vi "Generate Reference Waveforms.vi"(6 "reset phase":bool, 8 "error in (no error)":errorcluster, 11 "Generator in":refnum<class "Generator.lvclass">) -> (0 "error out":errorcluster, 1 "REF_Y":waveform(dbl)[](array[waveform]), 2 "REF_X":waveform(dbl)[](array[waveform]), 3 "Generator out":refnum<class "Generator.lvclass">, 4 "phase reset":bool)   [LabVIEW 2019, in "Generator.lvclass"]
uses:
  Generator.lvclass
  typedefs/REF.Channel--Cluster.ctl
  Generator.lvclass/Generator.ctl
  <vilib>/measure/NI_MABase.lvlib
  Waveform.Attributes/Waveform.Attributes.lvlib
panel:
  in  "Tab Control":enum32{"Page 1", "Graph"}(tab)
  out "sampling info":cluster{"Fs":dbl, "#s":dbl}={"Fs"=1000.0, "#s"=1000.0} {"Fs" format="%.2p"}
  out "REF Channels":T1[](array[typedef]) {"TC" min=1.0; "Phase" min=0.0001 format="%#_3p"; "Frequency" format="%.3g"; "Channel" min=1 max=10000 format="%.3g"}
  out "Waveform Graph":waveform(dbl)[](graph)
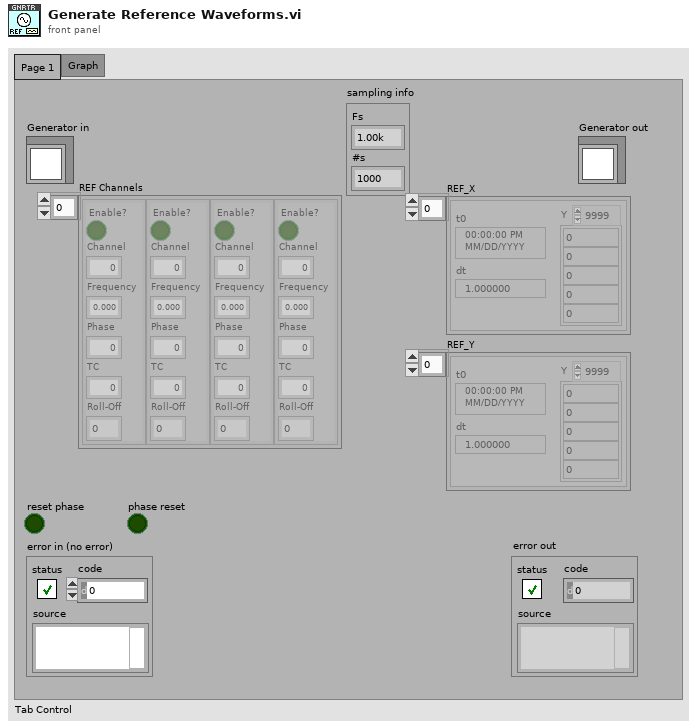
[diagram p1: front panel]
types:
  T1 = typedef "Generator.lvclass/REF.Channel--Cluster.ctl" = cluster{"Enable?":bool, "Channel":i32, "Frequency":dbl, "Phase":dbl, "TC":dbl, "Roll-Off":i32}
  T2 = typedef "Generator.lvclass/REF.Channel--Cluster--Array.ctl" = T1[]
  T3 = typedef "Generator.lvclass/Sampling--Cluster.ctl" = cluster{"Fs":dbl, "#s":dbl}
  T4 = enum16{"Sine Wave", "Triangle Wave", "Square Wave", "Sawtooth Wave"}
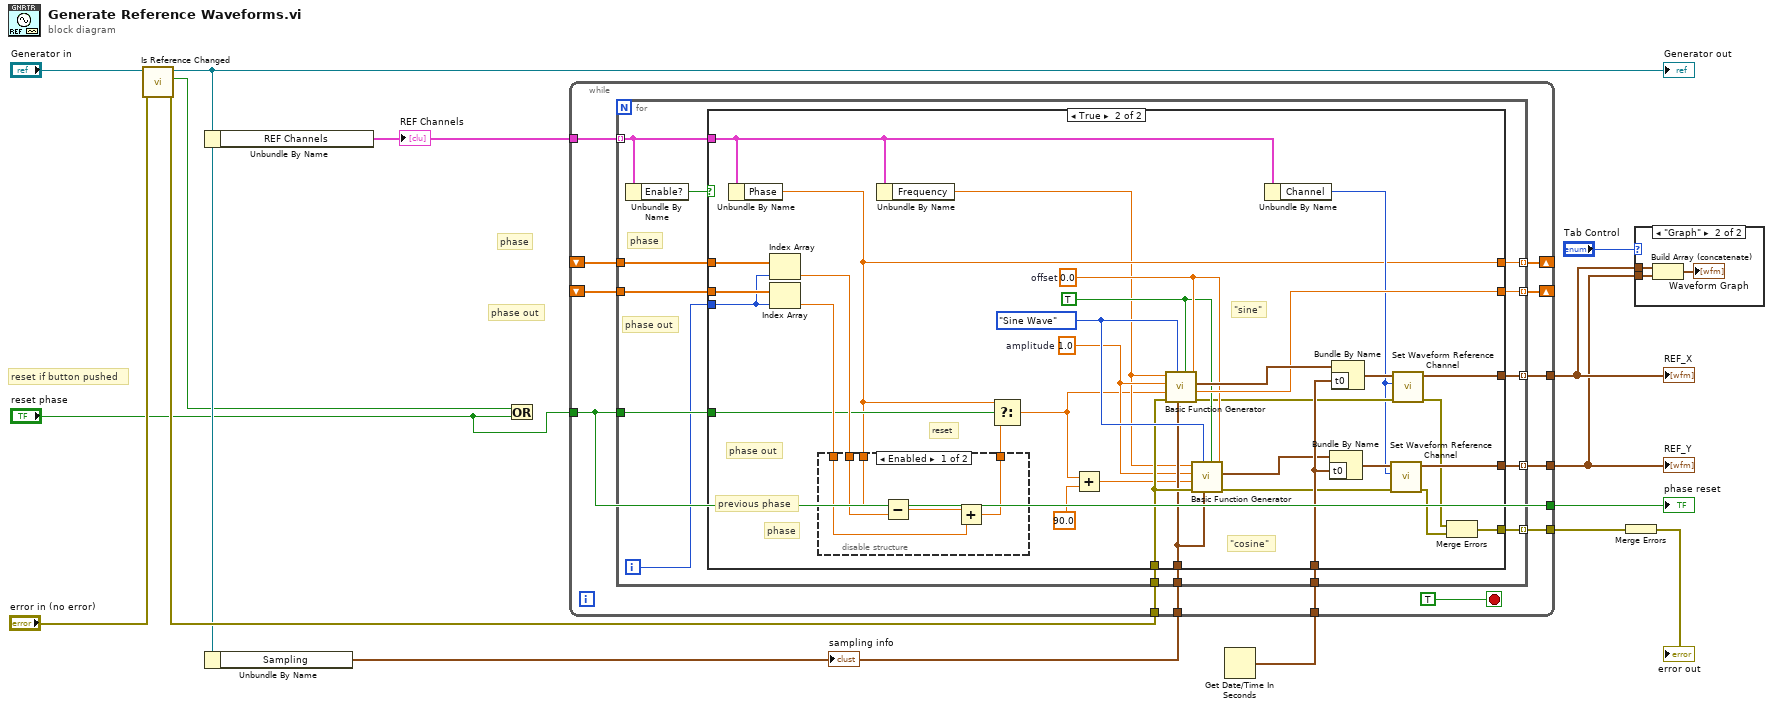
[diagram p0: block diagram]
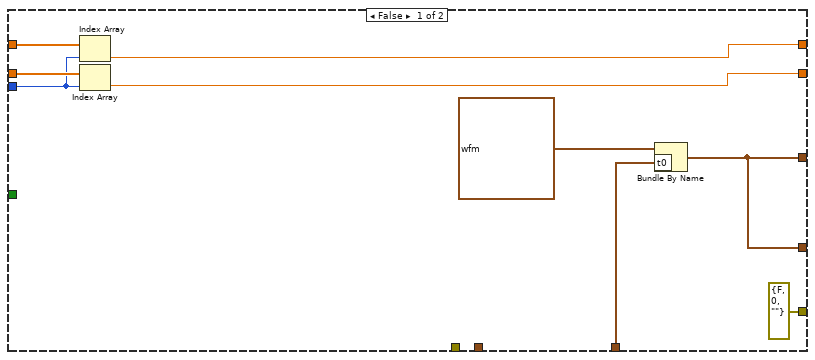
[diagram p2: hidden frame]
diagram:
  # "reset if button pushed"
  # "phase out"
  # "phase"
  n1 = call "Is Reference Changed.vi"("error in (no error)"="error in (no error)", "Generator in"="Generator in") -> ("error out"=w12:errorcluster, "REF frequency or phase changed?"=w3:bool, "Generator out"=w4:refnum<class "Generator.lvclass">)  [unwired: 7 in]
  "Generator out" <- w4
  n2 = Unbundle By Name(w4) -> ("REF Channels"=w1:T2)
  "REF Channels" <- w1
  n3 = Unbundle By Name(w4) -> ("Sampling"=w10:T3)
  "sampling info" <- w10
  n4 = Or(x=w3, y="reset phase") -> ()  [unwired: 1 out]
  n5 = Get Date/Time In Seconds() -> (seconds since 1Jan1904=w15:timestamp)
  n6 = while {
    tunnel: w10 -> [w28]
    shift-right: [w26] -> _
    shift-left: _ -> [w17]
    tunnel: w15 -> [w25]
    tunnel: w12 -> [w24]
    tunnel: w1 -> [w20]
    shift-right: [w23] -> _
    shift-left: _ -> [w21]
    tunnel: [w22] -> w9
    tunnel: [w19] -> w7
    tunnel: [w18] -> w6
    tunnel: [w16] -> w8
    tunnel: "reset phase" -> [w16]
    stop <- TRUE stop-if-true
    n7 = for {
      tunnel: w28 -> [w39]
      tunnel: [w42] -> w26 mode=indexing
      tunnel: w25 -> [w41]
      tunnel: w24 -> [w40]
      tunnel: w20 -> [w30] mode=indexing
      tunnel: w17 -> [w38]
      tunnel: [w31] -> w23 mode=indexing
      tunnel: w16 -> [w35]
      tunnel: w21 -> [w37]
      tunnel: [w36] -> w22 mode=indexing
      tunnel: [w34] -> w19 mode=indexing
      tunnel: [w33] -> w18 mode=indexing
      i -> [w32]
      # "phase out"
      # "phase"
      n8 = Unbundle By Name(w30) -> ("Enable?"=w29:bool)
      n9 = case shown="True" w29 {
        tunnel: [w44 w82] -> w42
        tunnel: w41 -> [w51 w81]
        tunnel: w40 -> [_ w77]
        tunnel: w39 -> [_ w76]
        tunnel: w38 -> [w47 w73]
        tunnel: w37 -> [w48 w72]
        tunnel: [errorcluster {"status"=FALSE, "code"=0, "source"=""} ("error IO") w71] -> w36
        tunnel: w35 -> [_ w67]
        tunnel: [w43 w65] -> w34
        tunnel: [w43 w63] -> w33
        tunnel: w32 -> [w46 w62]
        tunnel: [w45 w55] -> w31
        tunnel: w30 -> [_ w54]
        frame False {
          n10 = Index Array(array=w48, index=w46) -> (element=w45:dbl)
          n11 = Index Array(array=w47, index=w46) -> (element=w44:dbl)
          n12 = Bundle By Name(cluster=waveform(dbl) {"t0"=timestamp(0 s since 1904-01-01), "dt"=1.0, "Y"=[0.0]} ("Waveform out"), "t0"=w51) -> (w43:waveform(dbl))
        }
        frame True {
          w74 = TRUE ("reset signal")
          w78 = 0.0  # offset
          w79 = T4."Sine Wave" ("signal type")
          w75 = 1.0  # amplitude
          # "previous phase"
          # "phase"
          # "phase out"
          # "reset"
          # "\"cosine\""
          # "\"sine\""
          n13 = Unbundle By Name(w54) -> ("Phase"=w55:dbl)
          n14 = Index Array(array=w72, index=w62) -> (element=w70:dbl)
          n15 = Index Array(array=w73, index=w62) -> (element=w68:dbl)
          n16 = disable-structure shown="Enabled" {
            disable-tunnel: w55 -> [w89 _]
            disable-tunnel: w70 -> [w88 _]
            disable-tunnel: w68 -> [w85 w90]
            disable-tunnel: [w87 w90] -> w69
            frame Enabled {
              n17 = Subtract(x=w89, y=w88) -> (x-y=w86:dbl)
              n18 = Add(x=w86, y=w85) -> (x+y=w87:dbl)
            }
            frame Disabled {
            }
          }
          n19 = Unbundle By Name(w54) -> ("Frequency"=w53:dbl)
          n20 = Select(t=w55, s=w67, f=w69) -> (s? t:f=w52:dbl)
          n21 = Add(x=w52, y=90.0) -> (x+y=w56:dbl)
          n22 = call <vilib>:"Basic Function Generator.vi"("offset"=w78, "reset signal"=w74, "sampling info"=w76, "signal type"=w79, "error in (no error)"=w77, "phase"=w52, "amplitude"=w75, "frequency"=w53) -> ("error out"=w61:errorcluster, "phase out"=w82:dbl, "signal out"=w84:waveform(dbl))  [unwired: 1 in]
          n23 = call <vilib>:"Basic Function Generator.vi"("offset"=w78, "reset signal"=w74, "sampling info"=w76, "signal type"=w79, "error in (no error)"=w77, "phase"=w56, "amplitude"=w75, "frequency"=w53) -> ("error out"=w60:errorcluster, "signal out"=w80:waveform(dbl))  [unwired: 1 in, 1 out]
          n24 = Unbundle By Name(w54) -> ("Channel"=w57:i32)
          n25 = Bundle By Name(cluster=w80, "t0"=w81) -> (w64:waveform(dbl))
          n26 = Bundle By Name(cluster=w84, "t0"=w81) -> (w66:waveform(dbl))
          n27 = call "Set Waveform Reference Channel.vi"("error in (no error)"=w60, "Reference Ch"=w57, "Waveform in"=w64) -> ("error out"=w59:errorcluster, "Waveform out"=w63:waveform(dbl))  [unwired: 7 in]
          n28 = call "Set Waveform Reference Channel.vi"("error in (no error)"=w61, "Reference Ch"=w57, "Waveform in"=w66) -> ("error out"=w58:errorcluster, "Waveform out"=w65:waveform(dbl))  [unwired: 7 in]
          n29 = Merge Errors(w58, w59) -> (w71:errorcluster)
        }
      }
    }
  }
  "REF_X" <- w7
  "REF_Y" <- w6
  "phase reset" <- w8
  n30 = Merge Errors(w9) -> (→"error out":errorcluster)
  n31 = case shown="\"Graph\"" "Tab Control" {
    tunnel: w7 -> [_ w93]
    tunnel: w6 -> [_ w92]
    frame Default {
    }
    frame "Graph" {
      n32 = Build Array (concatenate)(w93, w92) -> (→"Waveform Graph":waveform(dbl)[])
    }
  }
